vi "2021 Advent puzzle 01b.vi"() -> ()   [LabVIEW 2021]
panel:
  out "array type (2D Dbl)":i32[][](array[numeric])
  out "sum":i16
  out "?":i16[](array[numeric])
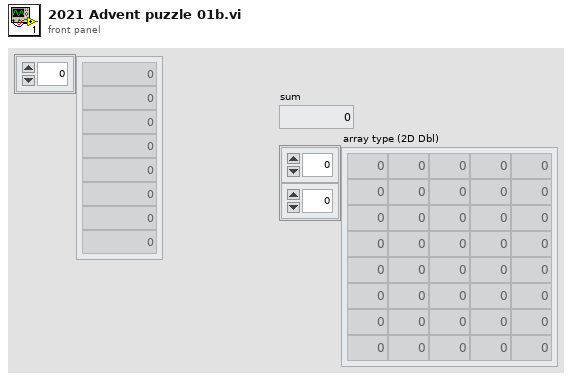
[diagram p1: front panel]
diagram:
  (unwired) "199  \n200    \n208  \n210\n200\n207\n240   \n269  \n260\n263  "
  # "find the number of increasing values of three succeeding values compared with a walking set"
  n1 = Spreadsheet String To Array(delimiter (Tab)="\n", format string="", spreadsheet string="188\n192\n193\n194\n192\n213\n214\n216\n219\n221\n222\n228\n231\n234\n239\n240\n252\n262\n267\n279\n278\n277\n279\n293\n309\n310\n312\n307\n308\n316\n320\n323\n335\n336\n343\n368\n357\n370\n377\n386\n387\n386\n402\n379\n393\n394\n403\n404\n405\n400\n421\n422\n423\n408\n409\n411\n408\n415\n417\n430\n439\n432\n459\n462\n463\n464\n466\n472\n485\n473\n488\n491\n492\n493\n496\n497\n501\n503\n516\n514\n513\n514\n517\n521\n522\n526\n548\n553\n560\n563\n565\n600\n601\n595\n596\n597\n599\n613\n630\n631\n635\n642\n648\n651\n654\n645\n653\n657\n676\n688\n711\n717\n718\n728\n735\n730\n733\n734\n737\n736\n738\n741\n749\n751\n752\n762\n765\n776\n779\n758\n743\n754\n759\n772\n773\n783\n790\n791\n783\n781\n784\n785\n791\n780\n789\n805\n792\n793\n797\n825\n...", array type (2D Dbl)=i32[] []) -> (array=w5:i32[])
  n2 = Array Size(array=w5) -> (size(s)=w4:i32)
  n3 = Array Subset(array=w5, index=0, length=3) -> (w9:i32[])
  n4 = Subtract(x=w4, y=3) -> (x-y=w3:i32)
  n5 = Add Array Elements(numeric array=w9) -> (sum=w8:i32)
  n6 = for {
    N: w3 -> [_]
    tunnel: w5 -> [w17]
    shift-right: [w20] -> _
    shift-left: w8 -> [w21]
    tunnel: [w18] -> w7 mode=indexing
    tunnel: [w16] -> w6 mode=indexing
    i -> [w24]
    n7 = Increment(x=w24) -> (x+1=w23:i32)
    n8 = Array Subset(array=w17, index=w23, length=3) -> (w16:i32[])
    n9 = Add Array Elements(numeric array=w16) -> (sum=w20:i32)
    n10 = Greater?(x=w20, y=w21) -> (0:w22:bool)
    n11 = Boolean To (0,1)(Boolean=w22) -> (0, 1=w18:i16)
  }
  "?" <- w7
  "array type (2D Dbl)" <- w6
  n12 = Add Array Elements(numeric array=w7) -> (sum=→"sum":i16)
